vi "FA_ConvertToINIConfig.vi"(8 "Error In":errorcluster, 11 "Config":T1) -> (0 "Error Out":errorcluster, 3 "XML String":string)   [LabVIEW 2014, in "FA_INI.lvlib"]
doc: "Converts a LabVIEW typedef describing an INI configuration into an XML string"
uses:
  FA_INI.lvlib
  FA_INIconfig.ctl
  FA_INI.ctl
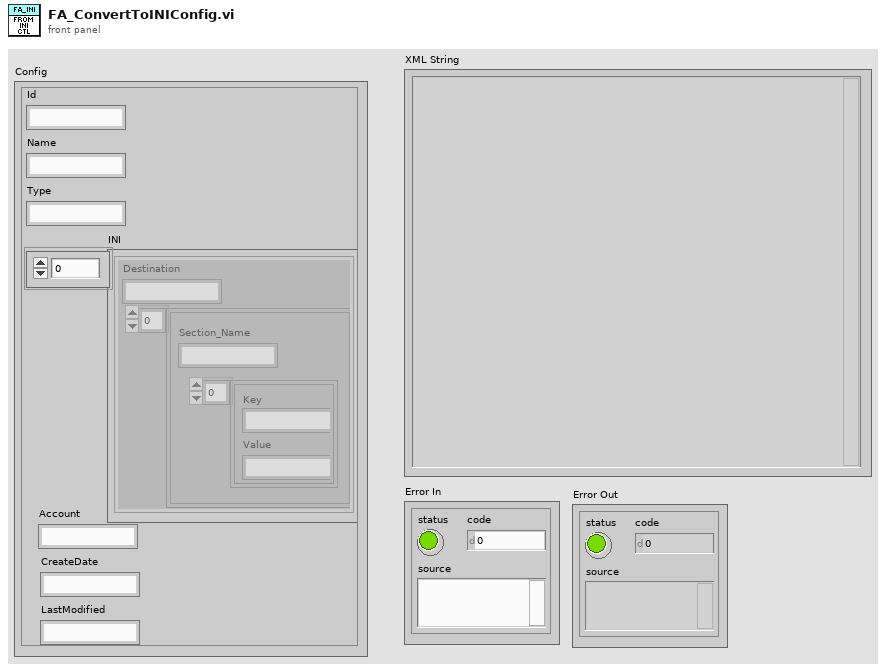
[diagram p1: front panel]
types:
  T1 = typedef "FA_INI.lvlib/FA_INIconfig.ctl" = cluster{"Id":string, "Name":string, "Type":string, "INI":T2, "Account":string, "CreateDate":string, "LastModified":string}
  T2 = typedef "FA_INI.ctl" = cluster{"Destination":string, "Section":cluster{"Section_Name":string, "Token":cluster{"Key":string, "Value":string}[]}[]}[]
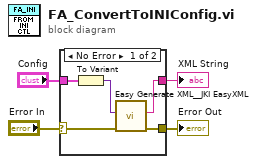
[diagram p0: block diagram]
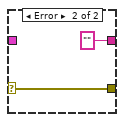
[diagram p2: hidden frame]
diagram:
  n1 = case shown="No Error" "Error In" {
    selector: "Error In" -> [w9 w11]
    tunnel: [w6 w11] -> w3
    tunnel: "Config" -> [w7 _]
    tunnel: [w5 "" ("XML String Out")] -> w1
    frame No Error {
      n2 = To Variant(anything=w7) -> (Variant=w8:variant)
      n3 = call <vilib>:"Easy Generate XML__JKI EasyXML.vi"("error in (no error)"=w9, "LabVIEW Data"=w8) -> ("error out"=w6:errorcluster, "XML String"=w5:string)  [unwired: 8 in]
    }
    frame Error {
    }
  }
  "XML String" <- w1
  "Error Out" <- w3
